vi "Program29.vi"() -> ()   [LabVIEW 2020]
panel:
  out "XY Graph 2":cluster{dbl[], dbl[]}[](graph)
  out "XY Graph":cluster{"X":dbl, "Y":dbl}[](graph)
  out "Waveform Graph 2":dbl[][](graph)
  out "Waveform Graph 1":dbl[](graph)
  out "Waveform Chart 2":cluster{dbl, dbl}(graph)
  out "Waveform Chart 1":dbl(graph)
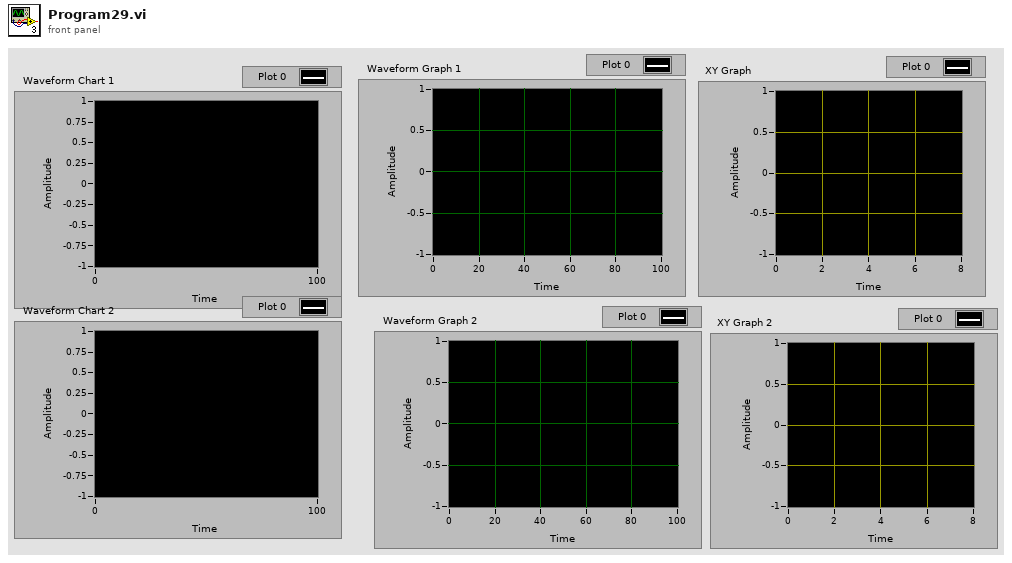
[diagram p1: front panel]
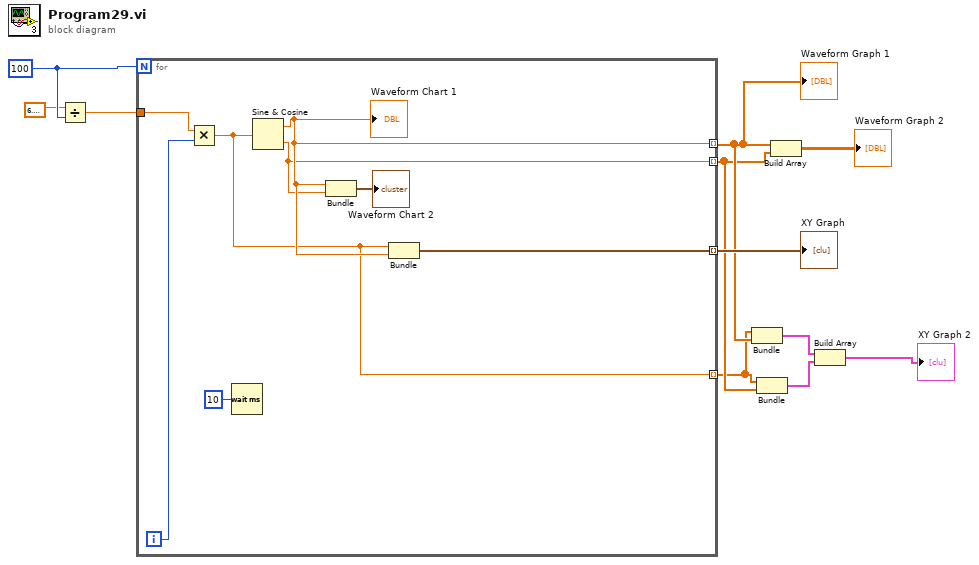
[diagram p0: block diagram]
diagram:
  w10 = 100
  n1 = Divide(x=6.283185307179586, y=w10) -> (x/y=w11:dbl)
  n2 = for {
    N: w10 -> [_]
    tunnel: w11 -> [w17]
    tunnel: [w15] -> w8 mode=indexing
    tunnel: [w14] -> w6 mode=indexing
    tunnel: [w13] -> w5 mode=indexing
    tunnel: [w12] -> w4 mode=indexing
    i -> [w18]
    n3 = Multiply(x=w17, y=w18) -> (x*y=w12:dbl)
    n4 = Wait (ms)(milliseconds to wait=u32 10) -> ()  [unwired: 1 out]
    n5 = Sine & Cosine(0:w12) -> (1:w14:dbl, 2:w13:dbl)
    "Waveform Chart 1" <- w14
    n6 = Bundle(w14, w13) -> (→"Waveform Chart 2":cluster{dbl, dbl})  [unwired: 1 in]
    n7 = Bundle(w12, w14) -> (w15:cluster{dbl, dbl})  [unwired: 1 in]
  }
  "Waveform Graph 1" <- w6
  "XY Graph" <- w8
  n8 = Bundle(w4, w6) -> (w3:cluster{dbl[], dbl[]})  [unwired: 1 in]
  n9 = Bundle(w4, w5) -> (w2:cluster{dbl[], dbl[]})  [unwired: 1 in]
  n10 = Build Array(w6, w5) -> (→"Waveform Graph 2":dbl[][])
  n11 = Build Array(w3, w2) -> (→"XY Graph 2":cluster{dbl[], dbl[]}[])
